vi "Word Example.vi"() -> ()   [LabVIEW 2017]
doc: "This example shows how to use the LabVIEW NPOI library to manipulate MS Word Files."
uses:
  LabVIEW NPOI/MS-Word/MS-Word.lvclass
  C:/Users/Neo/Desktop/Dev_Tools_BR/LabVIEW_NPOI/src/LabVIEW NPOI/Document/Document.lvclass
  LabVIEW NPOI/Document/Document.lvclass/Document.ctl
  LabVIEW NPOI/Document/Get FilePath.vi
  a6ef2128-b706-4ed5-9f9a-92b627d9699f.vi
  LabVIEW NPOI/Document/Read Table As String.vi
  LabVIEW NPOI/Document/Append Table (string).vi
  LabVIEW NPOI/Document/Append Table (double).vi
  LabVIEW NPOI/Document/Document.lvclass
panel:
  in  "print":bool
  in  "createDocumentBttn":bool
  in  "Text":string="Lorem ipsum dolor sit amet, consectetur adipiscing elit, sed do eiusmod tempor incididunt ut labore et dolore magna aliqua. Adipiscing bibendum est ultricies integer quis auctor elit sed vulputate. Volutpat consequat mauris nunc congue nisi vitae suscipit tellus. Eget arcu dictum varius duis at consectetur lorem donec massa. Morbi enim nunc faucibus a pellentesque sit. Risus ultricies tristique nulla aliquet enim tortor at. Sit amet consectetur adipiscing elit ut aliquam purus sit. Porta lorem mollis aliquam ut porttitor leo a diam. Odio aenean sed adipiscing diam donec adipiscing tristique risus. Nunc eget lorem dolor sed viverra ipsum nunc aliquet. Ultrices gravida dictum fusce ut. Mi eget mauris pharetra et ultrices. Ultrices dui sapien eget mi proin. Duis ut diam quam nulla porttitor massa id neque. Eu lobortis elementum nibh tellus molestie nunc non. Iaculis nunc sed augue lacus viverra. Enim sed faucibus turpis in eu. Quis viverra nibh cras pulvinar mattis. Auctor augue mauris augue neque gravida. Enim ut tellus elementum sagittis vitae."
  in  "addParagraphBttn":bool
  in  "HTML File Path":path
  in  "convertToHtml":bool
  out "Read Table Time":u32
  out "Add Table Time":u32
  in  "addImageBttn":bool
  out "Table Control":string[][](table)
  in  "readTableBttn":bool
  in  "#Columns":i32=100
  in  "#Rows":i32=2
  in  "tableType":enum32{"Strings", "Doubles"}(radio)
  in  "addTableBttn":bool
  out "FilePath":path
  in  "openDocumentBttn":bool
  in  "baseDocumentPath":path caption="Folder Path"
  in  "saveAsDocumentBttn":bool
  in  "saveDocumentBttn":bool
  in  "documentName":string="Book1.xlsx" caption="Name"
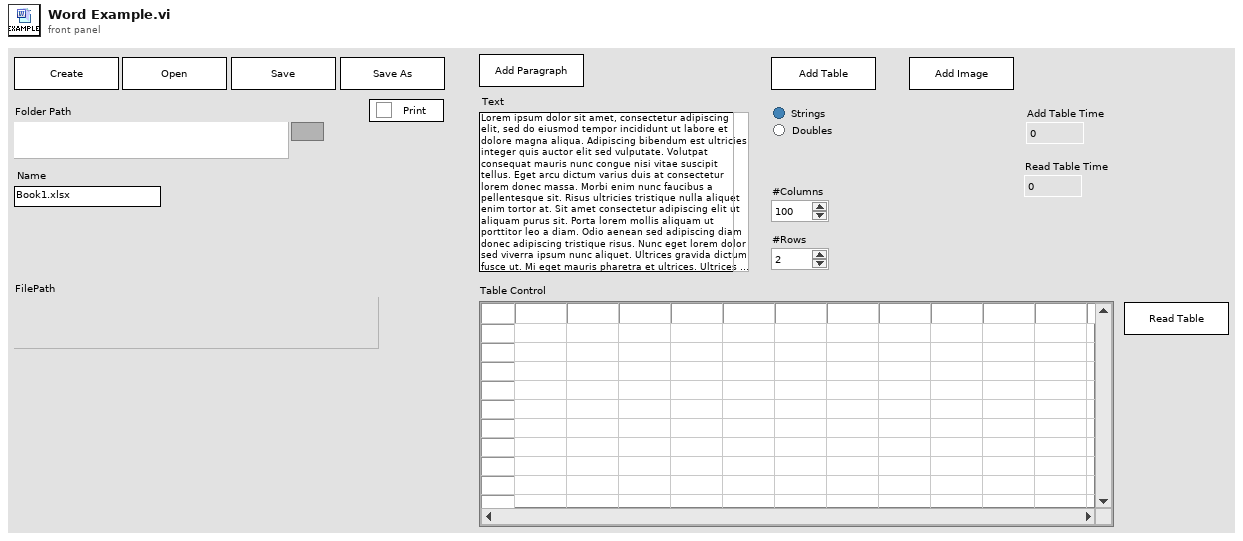
[diagram p1: front panel]
types:
  T1 = cluster{"documentObject":refnum<class "MS-Word.lvclass">, "documentPath":path, "documentName":string, "pageName":string, "styleName":string, "ctlRefs":refnum<vi>[]}
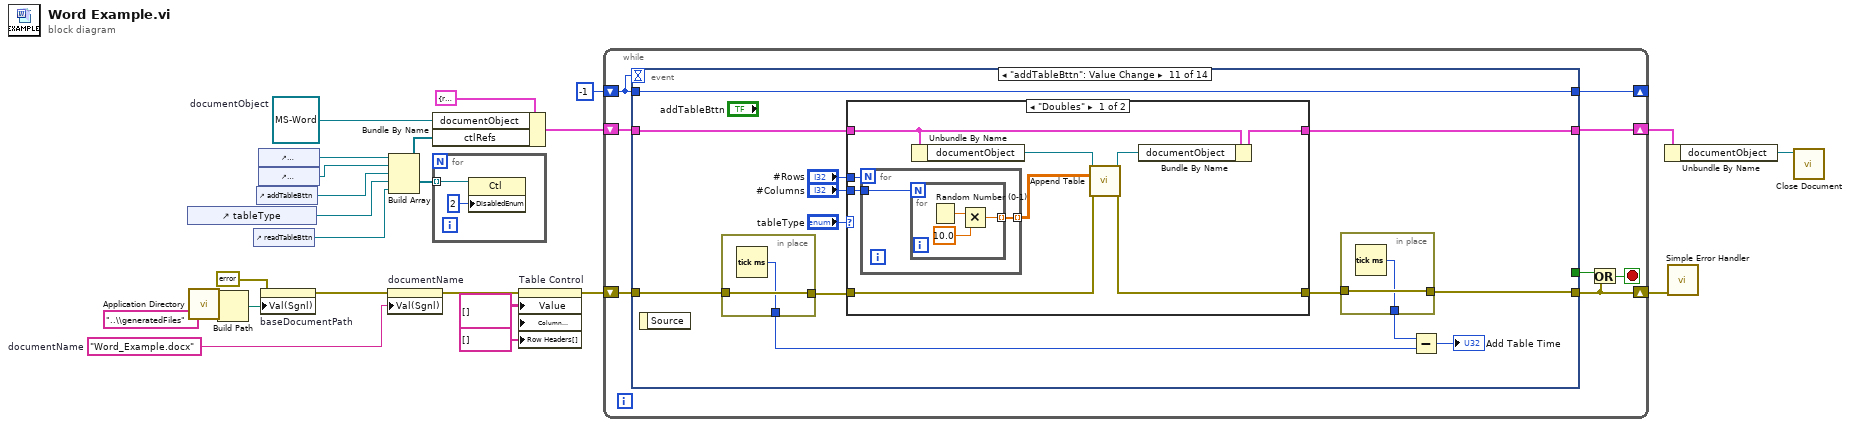
[diagram p0: block diagram]
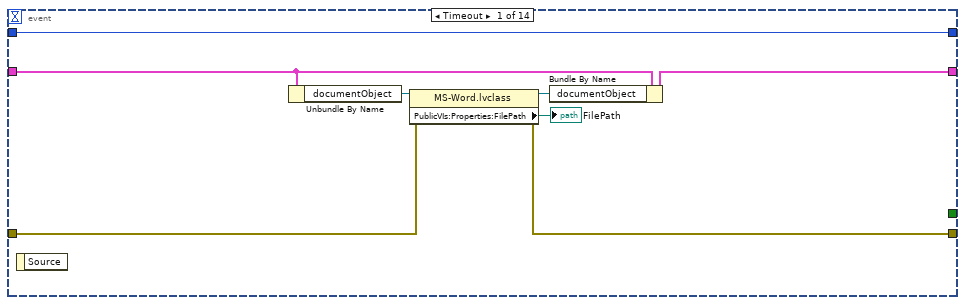
[diagram p2: hidden frame]
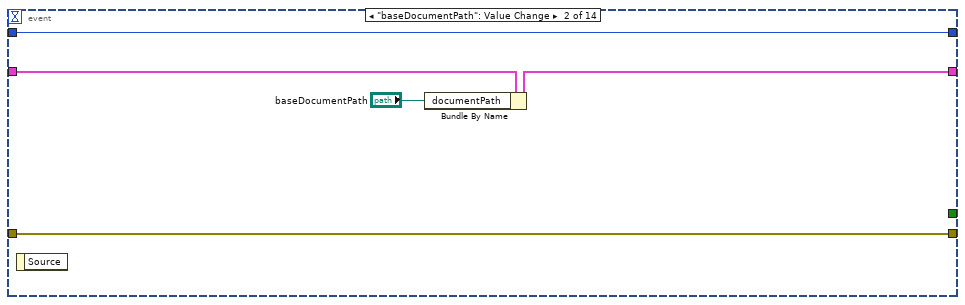
[diagram p3: hidden frame]
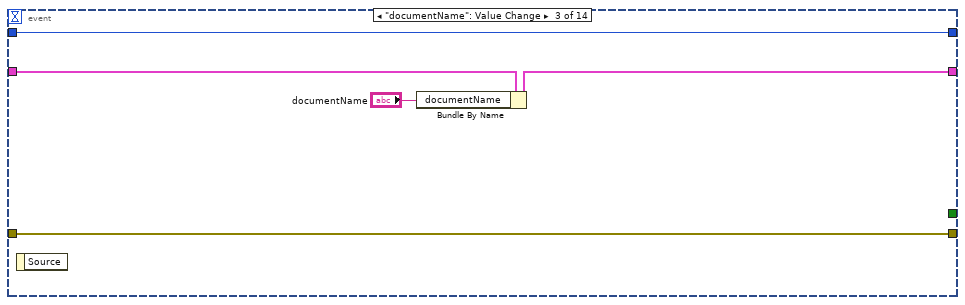
[diagram p4: hidden frame]
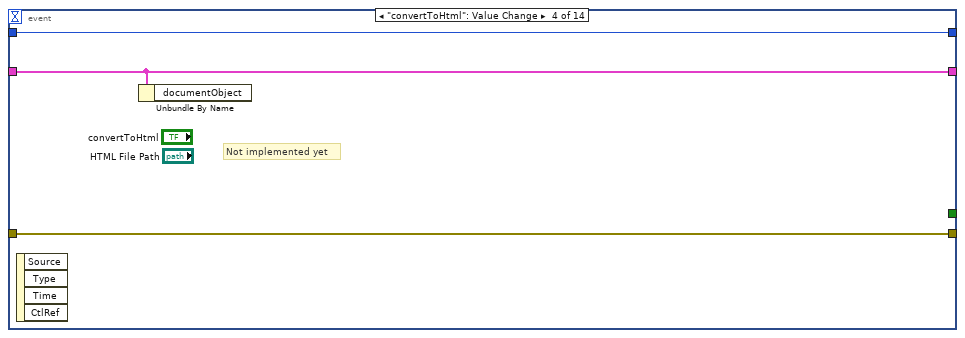
[diagram p5: hidden frame]
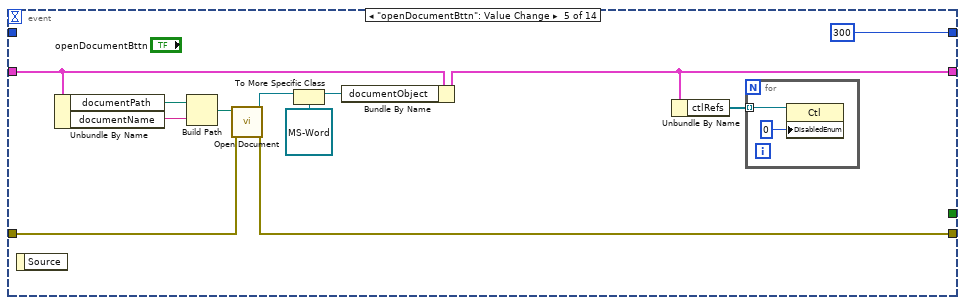
[diagram p6: hidden frame]
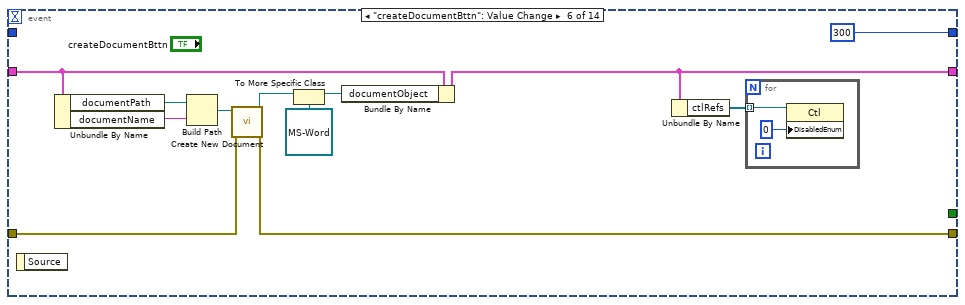
[diagram p7: hidden frame]
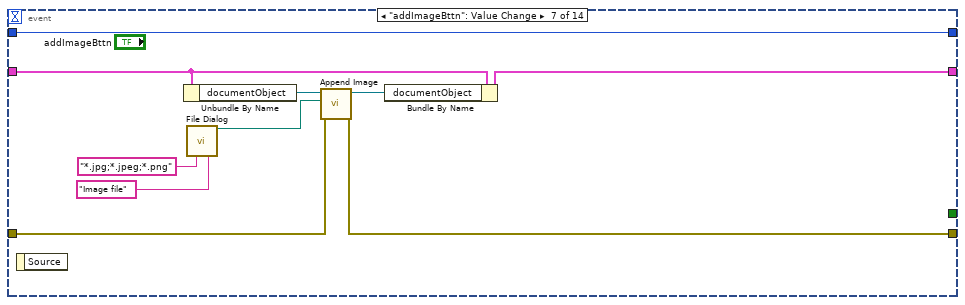
[diagram p8: hidden frame]
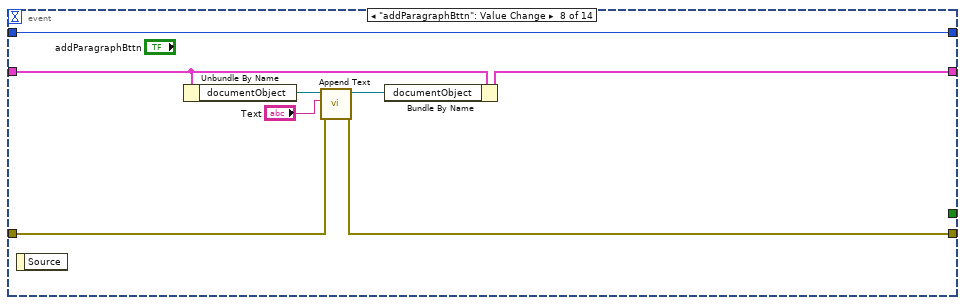
[diagram p9: hidden frame]
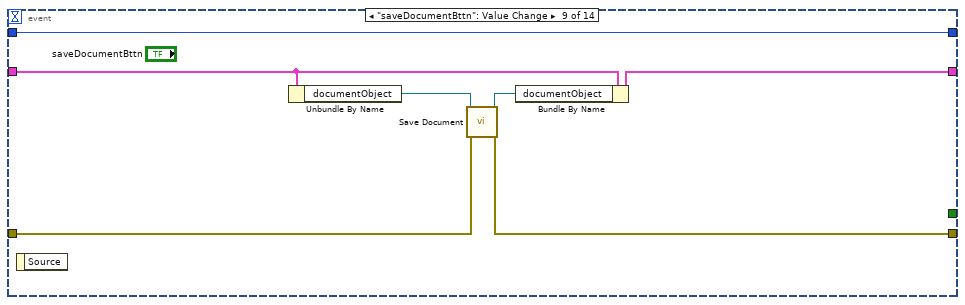
[diagram p10: hidden frame]
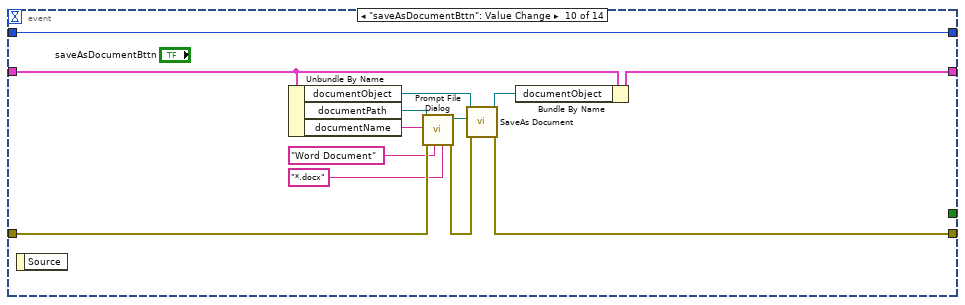
[diagram p11: hidden frame]
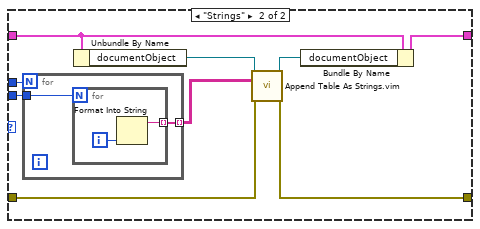
[diagram p12: hidden frame]
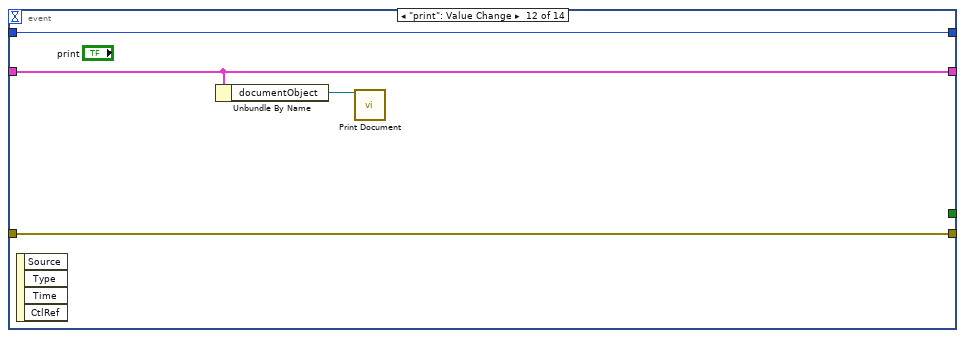
[diagram p13: hidden frame]
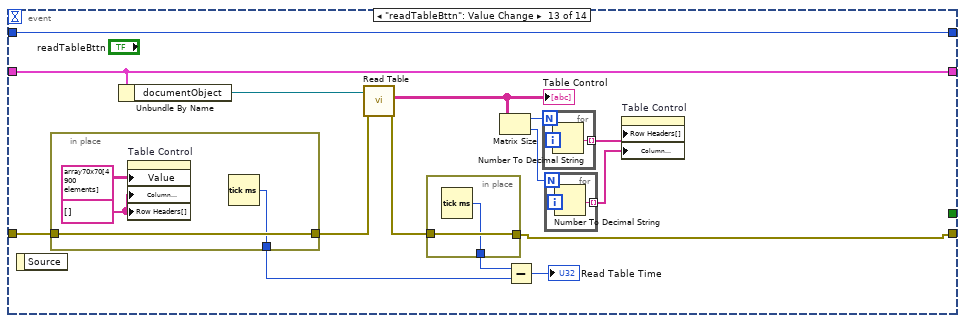
[diagram p14: hidden frame]
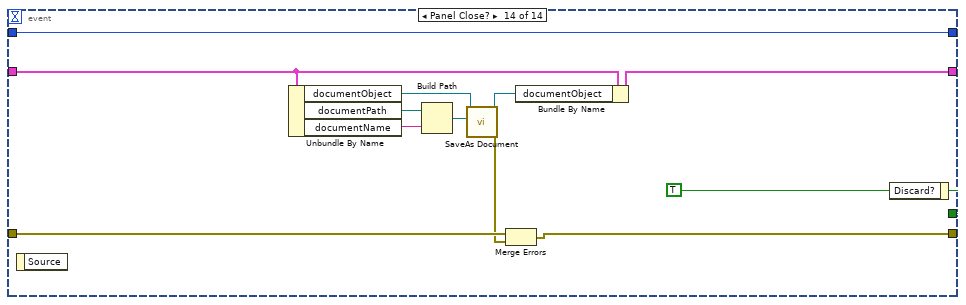
[diagram p15: hidden frame]
diagram:
  w8 = string[] [] ("Row Header Strings[]")
  w13 = "Word_Example.docx"  # documentName
  w17 = refnum<class "MS-Word.lvclass"> refnum  # documentObject
  n1 = control-ref of="tableType"() -> (w11:refnum<vi>)
  n2 = call <vilib>:"Application Directory.vi"() -> ("Application Directory"=w7:path)
  n3 = Build Path(base path=w7, name or relative path="..\\generatedFiles") -> (appended path=w4:path)
  n4 = control-ref of="readTableBttn"() -> (w10:refnum<vi>)
  n5 = control-ref of="addTableBttn"() -> (w12:refnum<vi>)
  n6 = control-ref of="saveDocumentBttn"() -> (w16:refnum<vi>)
  n7 = control-ref of="saveAsDocumentBttn"() -> (w15:refnum<vi>)
  n8 = property on="baseDocumentPath" class="Path"(error in=errorcluster {"status"=FALSE, "code"=0, "source"=""} ("error IO"), "Val(Sgnl)"=w4) -> (error out=w5:errorcluster)  [unwired: 1 in, 1 out]
  n9 = property on="documentName" class="Str"(error in=w5, "Val(Sgnl)"=w13) -> (error out=w3:errorcluster)  [unwired: 1 in, 1 out]
  n10 = Build Array(w16, w15, w12, w11, w10) -> (w14:refnum<vi>[])
  n11 = Bundle By Name(cluster=T1 {"documentObject"=refnum, "documentPath"=path "", "documentName"="", "pageName"="", "styleName"="Default", "ctlRefs"=[]}, "documentObject"=w17, "ctlRefs"=w14) -> (w23:T1)
  n12 = for {
    tunnel: w14 -> [w25] mode=indexing
    n13 = property class="Ctl"(reference=w25, "DisabledEnum"=u8 2) -> ()  [unwired: 1 in, 2 out]
  }
  n14 = property on="Table Control" class="Tbl (strict)"(error in=w3, "Value"=string[][] [] ("Table Control"), "Column Headers[]"=w8, "Row Headers[]"=w8) -> (error out=w1:errorcluster)  [unwired: 1 in, 1 out]
  n15 = while {
    shift-right: [w32] -> w20
    shift-left: w23 -> [w33]
    shift-right: [w30] -> w22
    shift-left: w1 -> [w31]
    shift-right: [w26] -> _
    shift-left: -1 -> [w27]
    stop <- w28 stop-if-true
    n16 = event shown="[10] \"addTableBttn\": Value Change" {
      selector: _ -> [_ _ _ _ _ _ _ _ _ _ _ _ _ _]
      dyn-events: _ -> [_ _ _ _ _ _ _ _ _ _ _ _ _ _]
      timeout: w27 -> [_ _ _ _ _ _ _ _ _ _ _ _ _ _]
      tunnel: [_ _ _ _ _ _ _ _ _ _ _ _ _ w198] -> w29
      tunnel: w33 -> [w41 w46 w51 w52 w66 w80 w91 w99 w107 w120 w128 w166 w182 w205]
      tunnel: [w34 w45 w50 w52 w61 w75 w87 w95 w105 w118 w133 w166 w182 w200] -> w32
      tunnel: [w37 w43 w48 w54 w55 w69 w88 w96 w103 w116 w124 w168 w172 w196] -> w30
      tunnel: w31 -> [w38 w43 w48 w54 w63 w77 w89 w97 w102 w114 w127 w168 w175 w197]
      tunnel: w27 -> [w35 w42 w47 w53 _ _ w92 w100 w101 w108 w132 w167 w183 w194]
      tunnel: [w35 w42 w47 w53 300 300 w92 w100 w101 w108 w132 w167 w183 w194] -> w26
      event Timeout {
        n17 = event-data() -> ()  [unwired: 1 in, 1 out]
        n18 = Unbundle By Name(w41) -> ("documentObject"=w40:refnum<class "MS-Word.lvclass">)
        n19 = property class="MS-Word.lvclass"(reference=w40, error in=w38) -> (reference out=w39:refnum<class "MS-Word.lvclass">, error out=w37:errorcluster, "PublicVIs:Properties:FilePath"=→"FilePath":path)
        n20 = Bundle By Name(cluster=w41, "documentObject"=w39) -> (w34:T1)
      }
      event "baseDocumentPath": Value Change {
        n21 = event-data() -> ()  [unwired: 1 in, 1 out]
        n22 = Bundle By Name(cluster=w46, "documentPath"="baseDocumentPath") -> (w45:T1)
      }
      event "documentName": Value Change {
        n23 = event-data() -> ()  [unwired: 1 in, 1 out]
        n24 = Bundle By Name(cluster=w51, "documentName"="documentName") -> (w50:T1)
      }
      event "convertToHtml": Value Change {
        # "Not implemented yet"
        n25 = event-data() -> ()  [unwired: 1 in, 4 out]
        n26 = Unbundle By Name(w52) -> ()  [unwired: 1 out]
      }
      event "openDocumentBttn": Value Change {
        n27 = event-data() -> ()  [unwired: 1 in, 1 out]
        n28 = Unbundle By Name(w66) -> ("documentPath"=w65:path, "documentName"=w64:string)
        n29 = Build Path(base path=w65, name or relative path=w64) -> (appended path=w59:path)
        n30 = call "Open Document.vi"("error in (no error)"=w63, "File Path"=w59) -> ("error out"=w55:errorcluster, "Document out"=w57:refnum<class "Document.lvclass">)  [unwired: 8 in]
        n31 = To More Specific Class(target class=refnum<class "MS-Word.lvclass"> refnum ("workbookObject"), reference=w57) -> (specific class reference=w56:refnum<class "MS-Word.lvclass">)  [unwired: 1 in, 1 out]
        n32 = Bundle By Name(cluster=w66, "documentObject"=w56) -> (w61:T1)
        n33 = Unbundle By Name(w61) -> ("ctlRefs"=w60:refnum<vi>[])
        n34 = for {
          tunnel: w60 -> [w68] mode=indexing
          n35 = property class="Ctl"(reference=w68, "DisabledEnum"=u8 0) -> ()  [unwired: 1 in, 2 out]
        }
      }
      event "createDocumentBttn": Value Change {
        n36 = event-data() -> ()  [unwired: 1 in, 1 out]
        n37 = Unbundle By Name(w80) -> ("documentPath"=w79:path, "documentName"=w78:string)
        n38 = Build Path(base path=w79, name or relative path=w78) -> (appended path=w73:path)
        n39 = call "Create New Document.vi"("error in (no error)"=w77, "File Path"=w73) -> ("error out"=w69:errorcluster, "Document out"=w71:refnum<class "Document.lvclass">)  [unwired: 8 in]
        n40 = To More Specific Class(target class=refnum<class "MS-Word.lvclass"> refnum ("workbookObject"), reference=w71) -> (specific class reference=w70:refnum<class "MS-Word.lvclass">)  [unwired: 1 in, 1 out]
        n41 = Bundle By Name(cluster=w80, "documentObject"=w70) -> (w75:T1)
        n42 = Unbundle By Name(w75) -> ("ctlRefs"=w74:refnum<vi>[])
        n43 = for {
          tunnel: w74 -> [w82] mode=indexing
          n44 = property class="Ctl"(reference=w82, "DisabledEnum"=u8 0) -> ()  [unwired: 1 in, 2 out]
        }
      }
      event "addImageBttn": Value Change {
        n45 = event-data() -> ()  [unwired: 1 in, 1 out]
        n46 = Unbundle By Name(w91) -> ("documentObject"=w90:refnum<class "MS-Word.lvclass">)
        n47 = call "File Dialog"("pattern (all files)"="*.jpg;*.jpeg;*.png", "pattern label"="Image file") -> ("selected path"=w85:path)  [unwired: 10 in, 3 out]
        n48 = call "Append Image.vi"("error in (no error)"=w89, "Image File Path"=w85, "Document in"=w90) -> ("error out"=w88:errorcluster, "Document out"=w86:refnum<class "MS-Word.lvclass">)  [unwired: 7 in]
        n49 = Bundle By Name(cluster=w91, "documentObject"=w86) -> (w87:T1)
      }
      event "addParagraphBttn": Value Change {
        n50 = event-data() -> ()  [unwired: 1 in, 1 out]
        n51 = Unbundle By Name(w99) -> ("documentObject"=w98:refnum<class "MS-Word.lvclass">)
        n52 = call "Append Text.vi"("error in (no error)"=w97, "Text"="Text", "Document in"=w98) -> ("error out"=w96:errorcluster, "Document out"=w94:refnum<class "MS-Word.lvclass">)  [unwired: 7 in]
        n53 = Bundle By Name(cluster=w99, "documentObject"=w94) -> (w95:T1)
      }
      event "saveDocumentBttn": Value Change {
        n54 = event-data() -> ()  [unwired: 1 in, 1 out]
        n55 = Unbundle By Name(w107) -> ("documentObject"=w106:refnum<class "MS-Word.lvclass">)
        n56 = call "Save Document.vi"("error in (no error)"=w102, "Document in"=w106) -> ("error out"=w103:errorcluster, "Document out"=w104:refnum<class "MS-Word.lvclass">)  [unwired: 8 in]
        n57 = Bundle By Name(cluster=w107, "documentObject"=w104) -> (w105:T1)
      }
      event "saveAsDocumentBttn": Value Change {
        n58 = event-data() -> ()  [unwired: 1 in, 1 out]
        n59 = Unbundle By Name(w120) -> ("documentObject"=w119:refnum<class "MS-Word.lvclass">, "documentPath"=w110:path, "documentName"=w109:string)
        n60 = call "Prompt File Dialog.vi"("pattern (all files)"="*.docx", "pattern label"="Word Document", "error in"=w114, "default name"=w109, "File Path"=w110) -> ("error out"=w113:errorcluster, "selected path"=w115:path)  [unwired: 5 in]
        n61 = call "SaveAs Document.vi"("error in (no error)"=w113, "File Path"=w115, "Document in"=w119) -> ("error out"=w116:errorcluster, "Document out"=w117:refnum<class "MS-Word.lvclass">)  [unwired: 7 in]
        n62 = Bundle By Name(cluster=w120, "documentObject"=w117) -> (w118:T1)
      }
      event "addTableBttn": Value Change {
        n63 = event-data() -> ()  [unwired: 1 in, 1 out]
        n64 = in-place {
          in-place-border: w127 -> [w137]
          in-place-border: [w137] -> w126
          in-place-border: [w136] -> w122
          n65 = Tick Count (ms)() -> (millisecond timer value=w136:u32)
        }
        n66 = case shown="\"Doubles\"" "tableType" {
          tunnel: w128 -> [w146 w160]
          tunnel: [w144 w158] -> w133
          tunnel: [w142 w156] -> w125
          tunnel: w126 -> [w141 w155]
          tunnel: "#Columns" -> [w138 w153]
          tunnel: "#Rows" -> [w139 w152]
          frame "Doubles" {
            n67 = for {
              N: w139 -> [_]
              tunnel: [w148] -> w140 mode=indexing
              tunnel: w138 -> [w147]
              n68 = for {
                N: w147 -> [_]
                tunnel: [w150] -> w148 mode=indexing
                n69 = Random Number (0-1)() -> (number: 0 to 1=w151:dbl)
                n70 = Multiply(x=w151, y=10.0) -> (x*y=w150:dbl)
              }
            }
            n71 = Unbundle By Name(w146) -> ("documentObject"=w145:refnum<class "MS-Word.lvclass">)
            n72 = call-poly "Append Table.vi"("Document in"=w145, "Table"=w140, "error in (no error)"=w141) -> ("Document out"=w143:refnum<class "MS-Word.lvclass">, "error out"=w142:errorcluster)  [unwired: 11 in]
            n73 = Bundle By Name(cluster=w146, "documentObject"=w143) -> (w144:T1)
          }
          frame "Strings" {
            n74 = for {
              N: w152 -> [_]
              tunnel: [w162] -> w154 mode=indexing
              tunnel: w153 -> [w161]
              n75 = for {
                N: w161 -> [_]
                tunnel: [w163] -> w162 mode=indexing
                i -> [w164]
                n76 = Format Into String(w164) -> (resulting string=w163:string)  [unwired: 3 in, 1 out]
              }
            }
            n77 = Unbundle By Name(w160) -> ("documentObject"=w159:refnum<class "MS-Word.lvclass">)
            n78 = call "Append Table As Strings.vim"("Document in"=w159, "Table"=w154, "error in (no error)"=w155) -> ("Document out"=w157:refnum<class "MS-Word.lvclass">, "error out"=w156:errorcluster)  [unwired: 11 in]
            n79 = Bundle By Name(cluster=w160, "documentObject"=w157) -> (w158:T1)
          }
        }
        n80 = in-place {
          in-place-border: w125 -> [w135]
          in-place-border: [w135] -> w124
          in-place-border: [w134] -> w123
          n81 = Tick Count (ms)() -> (millisecond timer value=w134:u32)
        }
        n82 = Subtract(x=w123, y=w122) -> (x-y=→"Add Table Time":u32)
      }
      event "print": Value Change {
        n83 = event-data() -> ()  [unwired: 1 in, 4 out]
        n84 = Unbundle By Name(w166) -> ("documentObject"=w165:refnum<class "MS-Word.lvclass">)
        n85 = call "Print Document.vi"("Document in"=w165) -> ()  [unwired: 9 in, 2 out]
      }
      event "readTableBttn": Value Change {
        n86 = event-data() -> ()  [unwired: 1 in, 1 out]
        n87 = in-place {
          in-place-border: w175 -> [w187]
          in-place-border: [w187] -> w174
          in-place-border: [w186] -> w170
          w189 = string[] [] ("Row Header Strings[]")
          n88 = property on="Table Control" class="Tbl (strict)"("Value"=string[][] array70x70[4900 elements] ("Table Control"), "Column Headers[]"=w189, "Row Headers[]"=w189) -> ()  [unwired: 2 in, 2 out]
          n89 = Tick Count (ms)() -> (millisecond timer value=w186:u32)
        }
        n90 = Unbundle By Name(w182) -> ("documentObject"=w181:refnum<class "MS-Word.lvclass">)
        n91 = call-poly "Read Table.vi"("error in (no error)"=w174, "Document in"=w181) -> ("error out"=w173:errorcluster, "Table As String"=w180:string[][])  [unwired: 7 in, 1 out]
        "Table Control" <- w180
        n92 = in-place {
          in-place-border: w173 -> [w185]
          in-place-border: [w185] -> w172
          in-place-border: [w184] -> w171
          n93 = Tick Count (ms)() -> (millisecond timer value=w184:u32)
        }
        n94 = Matrix Size(0:w180) -> (1:w179:i32, 2:w177:i32)
        n95 = Subtract(x=w171, y=w170) -> (x-y=→"Read Table Time":u32)
        n96 = for {
          N: w179 -> [_]
          tunnel: [w192] -> w178 mode=indexing
          i -> [w193]
          n97 = Number To Decimal String(number=w193) -> (decimal integer string=w192:string)  [unwired: 1 in]
        }
        n98 = for {
          N: w177 -> [_]
          tunnel: [w190] -> w176 mode=indexing
          i -> [w191]
          n99 = Number To Decimal String(number=w191) -> (decimal integer string=w190:string)  [unwired: 1 in]
        }
        n100 = property on="Table Control" class="Tbl (strict)"("Row Headers[]"=w178, "Column Headers[]"=w176) -> ()  [unwired: 2 in, 2 out]
      }
      event Panel Close? {
        w198 = TRUE ("Discard?")
        n101 = event-data() -> ()  [unwired: 1 in, 1 out]
        n102 = Unbundle By Name(w205) -> ("documentObject"=w202:refnum<class "MS-Word.lvclass">, "documentPath"=w204:path, "documentName"=w203:string)
        n103 = Build Path(base path=w204, name or relative path=w203) -> (appended path=w201:path)
        n104 = call "SaveAs Document.vi"("File Path"=w201, "Document in"=w202) -> ("error out"=w195:errorcluster, "Document out"=w199:refnum<class "MS-Word.lvclass">)  [unwired: 8 in]
        n105 = Merge Errors(w197, w195) -> (w196:errorcluster)
        n106 = Bundle By Name(cluster=w205, "documentObject"=w199) -> (w200:T1)
        n107 = event-data("Discard?"=w198) -> ()  [unwired: 1 in, 1 out]
      }
    }
    n108 = Or(x=w29, y=w30) -> (x .or. y?=w28:bool)
  }
  n109 = Unbundle By Name(w20) -> ("documentObject"=w19:refnum<class "MS-Word.lvclass">)
  n110 = call <vilib>:"Simple Error Handler.vi"("error in (no error)"=w22) -> ()  [unwired: 4 in, 5 out]
  n111 = call "Close Document.vi"("Document in"=w19) -> ()  [unwired: 10 in, 1 out]
